vi "SelectFileFolder(SubVI).vi"(0 "635nmSubFolder":path, 1 "Project Folder in":path, 2 "Wavelength String":string, 5 "780nmSubFolder":path, 7 "850nmSubFolder":path, 9 "name or relative path":string, 11 "error in":errorcluster) -> (6 "appended path":path, 15 "error out":errorcluster)   [LabVIEW 2017]
panel:
  out "Result Folder out":path
  # "Outputs"
  # "Inputs"
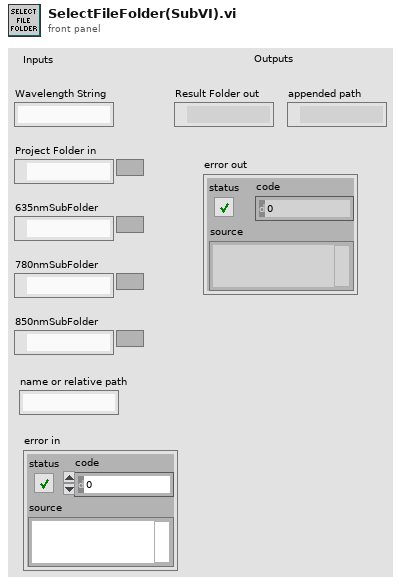
[diagram p1: front panel]
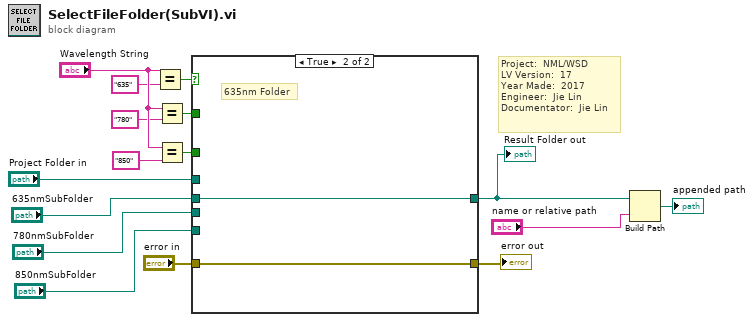
[diagram p0: block diagram]
diagram:
  # "Project:  NML/WSD \nLV Version:  17\nYear Made:  2017\nEngineer:  Jie Lin\nDocumentator:  Jie Lin"
  n1 = Equal?(x="Wavelength String", y="635") -> (x = y?=w10:bool)
  n2 = Equal?(x="Wavelength String", y="780") -> (x = y?=w12:bool)
  n3 = Equal?(x="Wavelength String", y="850") -> (x = y?=w14:bool)
  n4 = case shown="True" w10 {
    tunnel: "635nmSubFolder" -> [_ w38]
    tunnel: [w22 w38] -> w3
    tunnel: w12 -> [w24 _]
    tunnel: "780nmSubFolder" -> [w23 _]
    tunnel: w14 -> [w21 _]
    tunnel: "850nmSubFolder" -> [w20 _]
    tunnel: "Project Folder in" -> [w19 _]
    tunnel: "error in" -> [w18 w37]
    tunnel: [w17 w37] -> w4
    frame False {
      n5 = case shown="False" w24 {
        tunnel: w23 -> [_ w36]
        tunnel: [w28 w36] -> w22
        tunnel: w21 -> [w30 _]
        tunnel: w20 -> [w29 _]
        tunnel: w19 -> [w27 _]
        tunnel: w18 -> [w26 w35]
        tunnel: [w25 w35] -> w17
        frame False {
          n6 = case shown="False" w30 {
            tunnel: w29 -> [_ w34]
            tunnel: [w32 w34] -> w28
            tunnel: w27 -> [w32 _]
            tunnel: w26 -> [w31 w33]
            tunnel: [w31 w33] -> w25
            frame False {
              # "Project Folder"
            }
            frame True {
              # "850nm Folder"
            }
          }
        }
        frame True {
          # "780nm Folder"
        }
      }
    }
    frame True {
      # "635nm Folder"
    }
  }
  "Result Folder out" <- w3
  "error out" <- w4
  n7 = Build Path(base path=w3, name or relative path="name or relative path") -> (appended path=→"appended path":path)
